vi "Ticks Per Second to RPM.vi"(10 "Ticks per Rotation":dbl, 11 "Ticks Per Second":dbl) -> (3 "RPM":dbl)   [LabVIEW 2015]
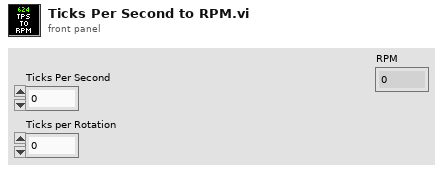
[diagram p1: front panel]
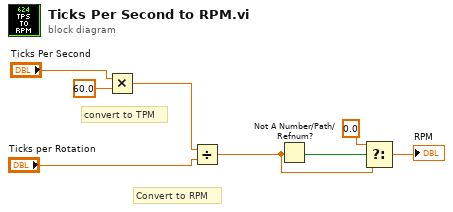
[diagram p0: block diagram]
diagram:
  # "Convert to RPM"
  # "convert to TPM"
  n1 = Multiply(x="Ticks Per Second", y=60.0) -> (x*y=w6:dbl)
  n2 = Divide(x=w6, y="Ticks per Rotation") -> (x/y=w2:dbl)
  n3 = Not A Number/Path/Refnum?(number/path/refnum=w2) -> (NaN/Path/Refnum?=w4:bool)
  n4 = Select(t=0.0, s=w4, f=w2) -> (s? t:f=→"RPM":dbl)
